vi "Write OT3.vi"(10 "OT3":refnum<class "OfficeTron3000.lvclass">, 11 "OT3IScan in":refnum<class "OT3IScan.lvclass">) -> (3 "OT3IScan out":refnum<class "OT3IScan.lvclass">)   [LabVIEW 2018, in "OfficeTron3000.lvlib" / "OT3IScan.lvclass"]
uses:
  OT3IScan.lvclass
  OfficeTron3000/OfficeTron3000.lvclass
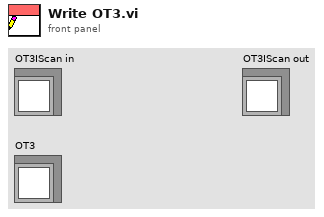
[diagram p1: front panel]
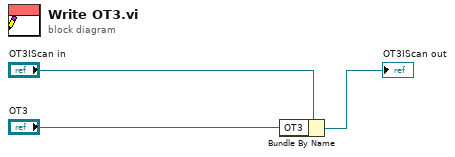
[diagram p0: block diagram]
diagram:
  n1 = Bundle By Name(cluster="OT3IScan in", "OT3"="OT3") -> (→"OT3IScan out":refnum<class "OT3IScan.lvclass">)
